vi "servo oscillation_rahul 2 (1).vi"() -> ()   [LabVIEW 2012]
uses:
  <vilib>/Motion/FlexMotion/FunctionsVIs/AxisResourceConfig.llb/Enable Axes (8 axes).flx
  <vilib>/Motion/FlexMotion/FunctionsVIs/Trajectory.llb/Load Accel/Decel in RPS/sec.flx
  <vilib>/Motion/FlexMotion/FunctionsVIs/StartStopMotion.llb/Blend Motion (8 axes).flx
  <vilib>/Motion/FlexMotion/FunctionsVIs/StartStopMotion.llb/Start Motion (8 axes).flx
  <vilib>/Motion/FlexMotion/FunctionsVIs/Trajectory.llb/Check Blend Complete Status (8 axes).flx
  <vilib>/Motion/FlexMotion/FunctionsVIs/Trajectory.llb/Check Move Complete Status (8 axes).flx
  <vilib>/Motion/FlexMotion/FunctionsVIs/StartStopMotion.llb/Stop Motion (8 axes).flx
  <vilib>/Analysis/NI_AALBase.lvlib
panel:
  out "Position":i32[](graph)
  in  "Choose Axis":T1
  in  "RUN":bool
  in  "Blend Factor":i16=-1 min=-1 max=16383
  in  "Velocity":dbl=1000.0 step=50.0 format="%.2f"
  in  "Acceleration":dbl=1000.0 min=0.0 format="%.2f"
  in  "Board ID":T2=1 min=1 max=32 step=1
  in  "samples per cycle":dbl=10.0
  in  "no of cycles":dbl=1.0
  in  "amplitude":dbl=15000.0 format="%0.2f"
  out "Current Position":dbl(slide)=37.0 scale=-20000.0..20000.0 scale format="%.2f"
  in  "STOP":bool
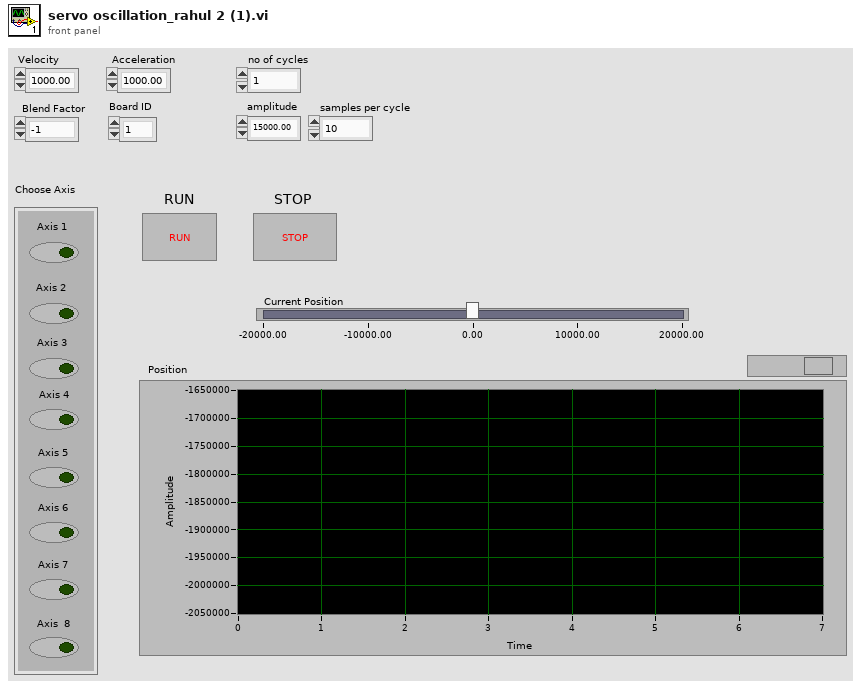
[diagram p1: front panel]
types:
  T1 = cluster{"Axis 1":bool, "Axis 2":bool, "Axis 3":bool, "Axis 4":bool, "Axis 5":bool, "Axis 6":bool, "Axis 7":bool, "Axis  8":bool}
  T2 = typedef "Board Id" = u8
  T3 = enum16{"Absolute Position", "Relative Position", "Velocity", "Relative to Cap Pos", "Modulus Position", "Absolute Contouring", "Relative Contouring"}
  T4 = typedef "Bd Id Out" = u8
  T5 = typedef "Resource Out (Enum).flx" = u16
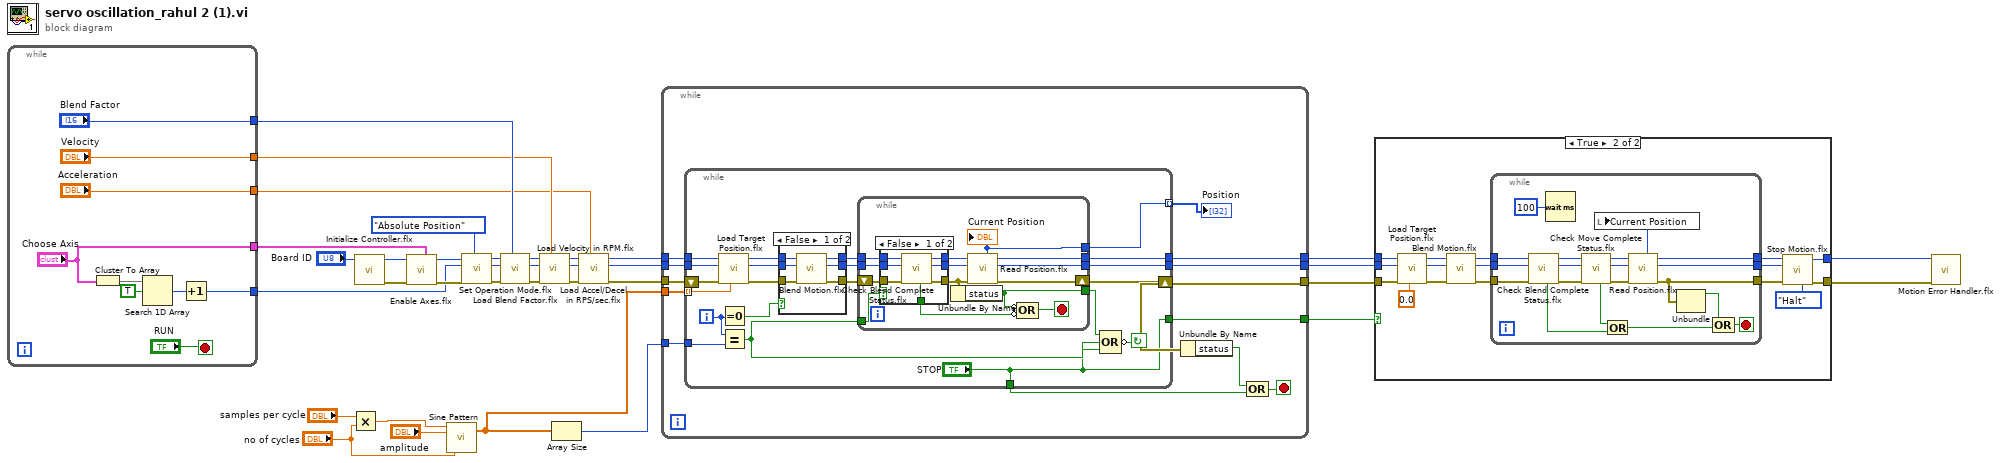
[diagram p0: block diagram]
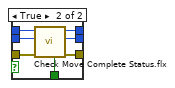
[diagram p3: hidden frame]
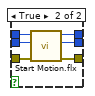
[diagram p4: hidden frame]
diagram:
  n1 = while {
    tunnel: ["Choose Axis"] -> w13
    tunnel: [w39] -> w10
    tunnel: ["Blend Factor"] -> w9
    tunnel: ["Velocity"] -> w8
    tunnel: ["Acceleration"] -> w7
    stop <- "RUN" stop-if-true
    n2 = Cluster To Array(cluster="Choose Axis") -> (array=w43:bool[])
    n3 = Search 1D Array(1D array=w43, element=TRUE) -> (index of element=w41:i32)  [unwired: 1 in]
    n4 = Increment(x=w41) -> (x+1=w39:i32)
  }
  n5 = Multiply(x="samples per cycle", y="no of cycles") -> (x*y=w18:dbl)
  n6 = call <vilib>:"Initialize Controller.flx"("Board ID"="Board ID") -> ("error out"=w15:errorcluster, "Bd ID Out"=w16:T4)  [unwired: 7 in]
  n7 = call-poly <vilib>:"Enable Axes.flx"("Axis Bitmap (Disabled)"=w13, "error in (no error)"=w15, "Board ID"=w16) -> ("error out"=w11:errorcluster, "Bd ID Out"=w12:T4)  [unwired: 5 in]
  n8 = call <vilib>:"Sine Pattern.vi"("cycles"="no of cycles", "amplitude"="amplitude", "samples"=w18) -> ("Sinusoidal Pattern"=w21:dbl[])  [unwired: 1 in, 1 out]
  n9 = call <vilib>:"Set Operation Mode.flx"("Position Mode (Absolute)"=T3."Absolute Position", "error in (no error)"=w11, "Axis or Vector Space"=w10, "Board ID"=w12) -> ("error out"=w25:errorcluster, "Resource Output"=w23:T5, "Bd ID Out"=w24:T4)  [unwired: 2 in]
  n10 = call <vilib>:"Load Blend Factor.flx"("Blend Factor (-1)"=w9, "error in (no error)"=w25, "Axis or Vector Space"=w23, "Board ID"=w24) -> ("error out"=w31:errorcluster, "Resource Output"=w33:T5, "Bd ID Out"=w34:T4)  [unwired: 3 in]
  n11 = call <vilib>:"Load Velocity in RPM.flx"("Velocity (500)"=w8, "error in (no error)"=w31, "Axis or Vector Space"=w33, "Board ID"=w34) -> ("error out"=w30:errorcluster, "Resource Output"=w32:T5, "Bd ID Out"=w35:T4)  [unwired: 3 in]
  n12 = Array Size(array=w21) -> (size(s)=w26:i32)
  n13 = call "Load Accel/Decel in RPS/sec.flx"("Value (200)"=w7, "error in (no error)"=w30, "Axis or Vector Space"=w32, "Board ID"=w35) -> ("error out"=w27:errorcluster, "Resource Output"=w28:T5, "Bd ID Out"=w29:T4)  [unwired: 3 in]
  n14 = while {
    tunnel: w29 -> [w57]
    tunnel: w28 -> [w56]
    tunnel: [w55] -> w4
    tunnel: [w54] -> w3
    tunnel: [w53] -> w1
    tunnel: [w49] -> w2
    tunnel: w27 -> [w52]
    tunnel: w26 -> [w51]
    tunnel: w21 -> [w50]
    stop <- w46 stop-if-true
    n15 = while {
      shift-left: w52 -> [w65]
      shift-right: [w63] -> w49
      tunnel: ["STOP"] -> w53
      tunnel: [w66] -> w54
      tunnel: [w67] -> w55
      tunnel: w50 -> [w69] mode=indexing
      tunnel: w51 -> [w68]
      tunnel: w56 -> [w73]
      tunnel: w57 -> [w72]
      tunnel: ["STOP"] -> w47
      tunnel: [w58] -> w45 mode=indexing
      i -> [w74]
      stop <- w61 continue-if-true
      n16 = call <vilib>:"Load Target Position.flx"("Target Position (0)"=w69, "error in (no error)"=w65, "Axis"=w73, "Board ID"=w72) -> ("error out"=w76:errorcluster, "Resource Output"=w77:T5, "Bd ID Out"=w78:T4)  [unwired: 3 in]
      n17 = Equal To 0?(x=w74) -> (x = 0?=w75:bool)
      n18 = Equal?(x=w74, y=w68) -> (x = y?=w62:bool)
      n19 = case shown="False" w75 {
        tunnel: w78 -> [w112 w118]
        tunnel: w77 -> [w111 w117]
        tunnel: w76 -> [w110 w116]
        tunnel: [w109 w115] -> w71
        tunnel: [w108 w114] -> w70
        tunnel: [w107 w113] -> w64
        frame False {
          n20 = call-poly <vilib>:"Blend Motion.flx"("error in (no error)"=w110, "Axis or Vector Space"=w111, "Board ID"=w112) -> ("error out"=w107:errorcluster, "Resource Output"=w108:T5, "Bd ID Out"=w109:T4)  [unwired: 3 in]
        }
        frame True {
          n21 = call-poly <vilib>:"Start Motion.flx"("error in (no error)"=w116, "Axis or Vector Space"=w117, "Board ID"=w118) -> ("error out"=w113:errorcluster, "Resource Output"=w114:T5, "Bd ID Out"=w115:T4)  [unwired: 3 in]
        }
      }
      n22 = while {
        tunnel: [w80] -> w60
        shift-left: w64 -> [w82]
        shift-right: [w81] -> w63
        tunnel: [w86] -> w66
        tunnel: [w87] -> w67
        tunnel: w62 -> [w84]
        tunnel: w70 -> [w90]
        tunnel: w71 -> [w91]
        tunnel: [w79] -> w58
        stop <- w92 stop-if-true
        n23 = case shown="False" w84 {
          tunnel: w91 -> [w99 w106]
          tunnel: w90 -> [w98 w105]
          tunnel: w82 -> [w97 w104]
          tunnel: [w96 w102] -> w89
          tunnel: [w95 w101] -> w88
          tunnel: [w94 w100] -> w83
          tunnel: [w93 w103] -> w85
          frame False {
            n24 = call-poly <vilib>:"Check Blend Complete Status.flx"("error in (no error)"=w97, "Axis or Vector Space"=w98, "Board ID"=w99) -> ("error out"=w93:errorcluster, "Resource Output"=w95:T5, "Bd ID Out"=w96:T4, "Blend Complete"=w94:bool)  [unwired: 3 in]
          }
          frame True {
            n25 = call-poly <vilib>:"Check Move Complete Status.flx"("error in (no error)"=w104, "Axis or Vector Space"=w105, "Board ID"=w106) -> ("error out"=w103:errorcluster, "Resource Output"=w101:T5, "Bd ID Out"=w102:T4, "Move Complete"=w100:bool)  [unwired: 3 in]
          }
        }
        n26 = Unbundle By Name(w85) -> ("status"=w80:bool)
        n27 = call <vilib>:"Read Position.flx"("error in (no error)"=w85, "Axis"=w88, "Board ID"=w89) -> ("error out"=w81:errorcluster, "Resource Output"=w86:T5, "Bd ID Out"=w87:T4, "Position"=w79:i32)  [unwired: 3 in]
        "Current Position" <- w79
        n28 = Compound Arithmetic op=OR(invert w80, invert w83) -> (w92:bool)
      }
      n29 = Compound Arithmetic op=OR(w60, "STOP", w62) -> (invert w61:bool)
    }
    "Position" <- w45
    n30 = Unbundle By Name(w49) -> ("status"=w48:bool)
    n31 = Compound Arithmetic op=OR(w48, w47) -> (w46:bool)
  }
  n32 = case shown="True" w1 {
    tunnel: [w120 w135] -> w6
    tunnel: [w119 w134] -> w5
    tunnel: w4 -> [w120 w123]
    tunnel: w3 -> [_ w122]
    tunnel: w2 -> [w119 w121]
    frame False {
    }
    frame True {
      n33 = call <vilib>:"Load Target Position.flx"("Target Position (0)"=0.0, "error in (no error)"=w121, "Axis"=w122, "Board ID"=w123) -> ("error out"=w132:errorcluster, "Resource Output"=w130:T5, "Bd ID Out"=w131:T4)  [unwired: 3 in]
      n34 = call-poly <vilib>:"Blend Motion.flx"("error in (no error)"=w132, "Axis or Vector Space"=w130, "Board ID"=w131) -> ("error out"=w128:errorcluster, "Resource Output"=w127:T5, "Bd ID Out"=w129:T4)  [unwired: 3 in]
      n35 = while {
        tunnel: w129 -> [w155]
        tunnel: w128 -> [w154]
        tunnel: w127 -> [w153]
        tunnel: [w151] -> w126
        tunnel: [w149] -> w125
        tunnel: [w150] -> w124
        stop <- w147 stop-if-true
        n36 = call-poly <vilib>:"Check Blend Complete Status.flx"("error in (no error)"=w154, "Axis or Vector Space"=w153, "Board ID"=w155) -> ("error out"=w144:errorcluster, "Resource Output"=w142:T5, "Bd ID Out"=w152:T4, "Blend Complete"=w139:bool)  [unwired: 3 in]
        n37 = Wait (ms)(milliseconds to wait=u32 100) -> ()  [unwired: 1 out]
        n38 = call-poly <vilib>:"Check Move Complete Status.flx"("error in (no error)"=w144, "Axis or Vector Space"=w142, "Board ID"=w152) -> ("error out"=w143:errorcluster, "Resource Output"=w141:T5, "Bd ID Out"=w145:T4, "Move Complete"=w140:bool)  [unwired: 3 in]
        n39 = Or(x=w140, y=w139) -> (x .or. y?=w138:bool)
        n40 = call <vilib>:"Read Position.flx"("error in (no error)"=w143, "Axis"=w141, "Board ID"=w145) -> ("error out"=w149:errorcluster, "Resource Output"=w150:T5, "Bd ID Out"=w151:T4, "Position"=w137:i32)  [unwired: 3 in]
        n41 = local write "Current Position"(w137) -> ()
        n42 = Unbundle(w149) -> ("status"=w148:bool)  [unwired: 2 out]
        n43 = Compound Arithmetic op=OR(w148, w138) -> (w147:bool)
      }
      n44 = call-poly <vilib>:"Stop Motion.flx"("Stop Type (Decel)"=enum16{"Decelerate", "Halt", "Kill"}."Halt", "error in (no error)"=w125, "Axis or Vector Space"=w124, "Board ID"=w126) -> ("error out"=w134:errorcluster, "Bd ID Out"=w135:T4)  [unwired: 3 in, 1 out]
    }
  }
  n45 = call <vilib>:"Motion Error Handler.flx"("Board ID"=w6, "error in (no error)"=w5) -> ()  [unwired: 9 in, 5 out]
